vi "HEWH RLT PRAT.vi"() -> ()   [LabVIEW 2016] (continued)
        n576 = local read "Temp Decline Complete D"() -> (w1181:bool)
        n577 = call "HEWH Temperature Decline.vi"("Error In"=w1182, "Station"="D", "Temp Decline Complete A"=w1181, "Draw Parameters Seq"=w1185) -> ("Error Out"=w1180:errorcluster, "Output States"=w1184:string)  [unwired: 5 in, 1 out]
        n578 = call <vilib>:"Add State(s) to Queue__jki_lib_state_machine.vi"("State(s) in Front (\"\")"=w1184, "State(s) in (\"\")"=w1189) -> ("States Out"=w1188:string)  [unwired: 13 in]
      }
      frame "Set Draw Station" {
        n579 = case shown="\"D\"" w1197 {
          tunnel: w1196 -> [w1217 w1233 w1251 w1268]
          tunnel: [w1216 w1234 w1250 w1267] -> w1198
          tunnel: w1194 -> [w1213 w1230 w1245 w1264]
          tunnel: w1193 -> [w1210 _ _ _]
          tunnel: w1192 -> [_ w1227 _ _]
          tunnel: w1191 -> [_ _ w1244 _]
          tunnel: w1190 -> [_ _ _ w1261]
          frame "A", Default {
            n580 = Unbundle By Name(w1210) -> ("GEA2 Reference Out"=w1219:refnum<k24>, "GEA2 Event Registration"=w1218:refnum<event-registration>)
            n581 = Unbundle By Name(w1213) -> ("Draw Parameters Seq"=w1212:T41)
            n582 = Unbundle By Name(w1212) -> ("Station A.Mode Setting"=w1211:T15)
            n583 = call "HEWH_DSM_CMD.vi"("Heating Mode"=w1211, "GEA2 Commands and Requests"=GEA2_Commands."CMD_UPDATE_MODE") -> ("Input Data"=w1214:T74)  [unwired: 7 in, 1 out]
            n584 = for {
              N: 5 -> [_]
              tunnel: w1219 -> [w1225]
              tunnel: w1218 -> [w1224]
              tunnel: w1214 -> [w1221]
              shift-right: [w1222] -> w1216
              shift-left: w1217 -> [w1223]
              n585 = call "GEA2 Send and Receive Message.vi"("GEA2 Reference In"=w1225, "Input Data"=w1221, "GEA2 Event Registration"=w1224, "Error In"=w1223) -> ("Error Out"=w1222:errorcluster)  [unwired: 6 in, 5 out]
              n586 = Wait Until Next ms Multiple(millisecond multiple=u32 100) -> ()  [unwired: 1 out]
            }
          }
          frame "B" {
            n587 = Unbundle By Name(w1230) -> ("Draw Parameters Seq"=w1229:T41)
            n588 = Unbundle By Name(w1227) -> ("GEA2 Reference Out"=w1236:refnum<k24>, "GEA2 Event Registration"=w1235:refnum<event-registration>)
            n589 = Unbundle By Name(w1229) -> ("Station B.Mode Setting"=w1228:T15)
            n590 = call "HEWH_DSM_CMD.vi"("Heating Mode"=w1228, "GEA2 Commands and Requests"=GEA2_Commands."CMD_UPDATE_MODE") -> ("Input Data"=w1231:T74)  [unwired: 7 in, 1 out]
            n591 = for {
              N: 5 -> [_]
              tunnel: w1236 -> [w1242]
              tunnel: w1235 -> [w1241]
              tunnel: w1231 -> [w1238]
              shift-right: [w1240] -> w1234
              shift-left: w1233 -> [w1239]
              n592 = call "GEA2 Send and Receive Message.vi"("GEA2 Reference In"=w1242, "Input Data"=w1238, "GEA2 Event Registration"=w1241, "Error In"=w1239) -> ("Error Out"=w1240:errorcluster)  [unwired: 6 in, 5 out]
              n593 = Wait Until Next ms Multiple(millisecond multiple=u32 100) -> ()  [unwired: 1 out]
            }
          }
          frame "C" {
            n594 = Unbundle By Name(w1245) -> ("Draw Parameters Seq"=w1247:T41)
            n595 = Unbundle By Name(w1244) -> ("GEA2 Reference Out"=w1253:refnum<k24>, "GEA2 Event Registration"=w1252:refnum<event-registration>)
            n596 = Unbundle By Name(w1247) -> ("Station C.Mode Setting"=w1246:T15)
            n597 = call "HEWH_DSM_CMD.vi"("Heating Mode"=w1246, "GEA2 Commands and Requests"=GEA2_Commands."CMD_UPDATE_MODE") -> ("Input Data"=w1248:T74)  [unwired: 7 in, 1 out]
            n598 = for {
              N: 5 -> [_]
              tunnel: w1253 -> [w1259]
              tunnel: w1252 -> [w1258]
              tunnel: w1248 -> [w1255]
              shift-right: [w1256] -> w1250
              shift-left: w1251 -> [w1257]
              n599 = call "GEA2 Send and Receive Message.vi"("GEA2 Reference In"=w1259, "Input Data"=w1255, "GEA2 Event Registration"=w1258, "Error In"=w1257) -> ("Error Out"=w1256:errorcluster)  [unwired: 6 in, 5 out]
              n600 = Wait Until Next ms Multiple(millisecond multiple=u32 100) -> ()  [unwired: 1 out]
            }
          }
          frame "D" {
            n601 = Unbundle By Name(w1264) -> ("Draw Parameters Seq"=w1263:T41)
            n602 = Unbundle By Name(w1261) -> ("GEA2 Reference Out"=w1270:refnum<k24>, "GEA2 Event Registration"=w1269:refnum<event-registration>)
            n603 = Unbundle By Name(w1263) -> ("Station D.Mode Setting"=w1262:T15)
            n604 = call "HEWH_DSM_CMD.vi"("Heating Mode"=w1262, "GEA2 Commands and Requests"=GEA2_Commands."CMD_UPDATE_MODE") -> ("Input Data"=w1265:T74)  [unwired: 7 in, 1 out]
            n605 = for {
              N: 5 -> [_]
              tunnel: w1270 -> [w1276]
              tunnel: w1269 -> [w1275]
              tunnel: w1265 -> [w1272]
              shift-right: [w1273] -> w1267
              shift-left: w1268 -> [w1274]
              n606 = call "GEA2 Send and Receive Message.vi"("GEA2 Reference In"=w1276, "Input Data"=w1272, "GEA2 Event Registration"=w1275, "Error In"=w1274) -> ("Error Out"=w1273:errorcluster)  [unwired: 6 in, 5 out]
              n607 = Wait Until Next ms Multiple(millisecond multiple=u32 100) -> ()  [unwired: 1 out]
            }
          }
        }
        n608 = for {
          N: 10 -> [_]
          tunnel: w1197 -> [w1204]
          shift-right: [w1206] -> w1199
          shift-left: w1198 -> [w1205]
          n609 = Wait Until Next ms Multiple(millisecond multiple=u32 100) -> ()  [unwired: 1 out]
          n610 = call "UTILITY String Notifier.vi"("Status"=UTILITY_Notifier."Set", "error in (no error)"=w1205, "Set Status"=w1204, "name (unnamed)"="Draw Station") -> ("error out"=w1206:errorcluster)  [unwired: 6 in, 1 out]
        }
        n611 = call <vilib>:"Add State(s) to Queue__jki_lib_state_machine.vi"("State(s) in (\"\")"=w1202) -> ("States Out"=w1201:string)  [unwired: 14 in]
        "Draw Station" <- w1197
      }
      frame "-------Dispense Algorithm--------" {
        n612 = call <vilib>:"Add State(s) to Queue__jki_lib_state_machine.vi"("State(s) in (\"\")"=w1281) -> ("States Out"=w1280:string)  [unwired: 14 in]
      }
      frame "Dispense Gallons" {
        n613 = Unbundle By Name(w1311) -> ("Current Cond A"=w1286:T1, "Current Cond B"=w1285:T1, "Current Cond C"=w1284:T1, "Current Cond D"=w1283:T1, "Draw Parameters Seq.Station A.Flow Rate (GPM)"=→"GPM Target (Station A)":dbl, "Draw Parameters Seq.Station B.Flow Rate (GPM)"=→"GPM Target (Station B)":dbl, "Draw Parameters Seq.Station C.Flow Rate (GPM)"=→"GPM Target (Station C)":dbl, "Draw Parameters Seq.Station D.Flow Rate (GPM)"=→"GPM Target (Station D)":dbl, "Draw Parameters Seq.Station A.Temperature (F)"=→"Degree Setting( Station A)":dbl, "Draw Parameters Seq.Station B.Temperature (F)"=→"Degree Setting( Station B)":dbl, "Draw Parameters Seq.Station C.Temperature (F)"=→"Degree Setting( Station C)":dbl, "Draw Parameters Seq.Station D.Temperature (F)"=→"Degree Setting( Station D)":dbl, "Draw Parameters Seq.Station D.Condition Value #1"=w1296:dbl, "Draw Parameters Seq.Station C.Condition Value #1"=w1297:dbl, "Draw Parameters Seq.Station B.Condition Value #1"=w1298:dbl, "Draw Parameters Seq.Station A.Condition Value #1"=w1299:dbl, "Draw Parameters Seq.Station A.Terminate Condition"=w1295:T16, "Draw Parameters Seq.Station B.Terminate Condition"=w1294:T16, "Draw Parameters Seq.Station C.Terminate Condition"=w1293:T16, "Draw Parameters Seq.Station D.Terminate Condition"=w1291:T16, "Draw Parameters Seq"=w1292:T41)
        n614 = call "HEWH Update Draw Amount Display.vi"("Terminate Condition A"=w1295, "Terminate Condition B"=w1294, "Terminate Condition C"=w1293, "Terminate Condition D"=w1291, "Error In"=w1301, "Gallons to Draw A"=w1299, "Gallons to Draw B"=w1298, "Gallons to Draw C"=w1297, "Gallons to Draw D"=w1296) -> ("Draw Amount (Station A)"=→"Draw Amount (Station A)":dbl, "Draw Amount (Station B)"=→"Draw Amount (Station B)":dbl, "Draw Amount (Station C)"=→"Draw Amount (Station C)":dbl, "Draw Amount (Station D)"=→"Draw Amount (Station D)":dbl, "Error Out"=w1300:errorcluster)  [unwired: 6 in]
        n615 = flat-sequence {
          tunnel: [w1329] -> w1317
          tunnel: w1300 -> [w1328]
          tunnel: [w1328] -> w1316
          tunnel: w1314 -> [w1327]
          tunnel: [w1327] -> w1313
          tunnel: w1292 -> [w1326]
          tunnel: [w1325] -> w1310
          tunnel: w1286 -> [w1324]
          tunnel: w1285 -> [w1323]
          tunnel: w1284 -> [w1322]
          tunnel: w1283 -> [w1321]
          tunnel: [w1320] -> w1282
          tunnel: w1317 -> [w1361]
          tunnel: [w1365] -> w1315
          tunnel: w1316 -> [w1367]
          tunnel: w1313 -> [w1368]
          tunnel: [w1366] -> w1312
          tunnel: w1310 -> [w1360]
          tunnel: w1282 -> [w1359]
          frame #0 {
            n616 = local read "Draw Station"() -> (w1330:string)
            n617 = case shown="\"D\"" w1330 {
              tunnel: [Station_ID_Selector."A" ("Station ID") Station_ID_Selector."B" ("Station ID") Station_ID_Selector."C" ("Station ID") Station_ID_Selector."D" ("Station ID")] -> w1329
              tunnel: w1326 -> [w1336 w1343 w1350 w1355]
              tunnel: [w1334 w1342 w1349 w1358] -> w1325
              tunnel: w1324 -> [w1331 _ _ _]
              tunnel: w1323 -> [_ w1338 _ _]
              tunnel: w1322 -> [_ _ w1345 _]
              tunnel: w1321 -> [_ _ _ w1352]
              tunnel: [w1331 w1338 w1345 w1352] -> w1320
              frame "A", Default {
                n618 = Unbundle By Name(w1336) -> ("Station A"=w1335:T14)
                n619 = local read "Use Last Start Condition A?"() -> (w1333:bool)
                n620 = local read "Station A Test Sequence"() -> (w1332:T14[])
                n621 = call "HEWH Set Draw Station.vi"("Use Last Start Condition?"=w1333, "Station"=w1335, "Station Test Sequence"=w1332) -> ("Station Set"=w1334:T14)  [unwired: 7 in, 1 out]
              }
              frame "B" {
                n622 = local read "Use Last Start Condition B?"() -> (w1339:bool)
                n623 = local read "Station B Test Sequence"() -> (w1341:T14[])
                n624 = Unbundle By Name(w1343) -> ("Station B"=w1340:T14)
                n625 = call "HEWH Set Draw Station.vi"("Use Last Start Condition?"=w1339, "Station"=w1340, "Station Test Sequence"=w1341) -> ("Station Set"=w1342:T14)  [unwired: 7 in, 1 out]
              }
              frame "C" {
                n626 = local read "Station C Test Sequence"() -> (w1348:T14[])
                n627 = local read "Use Last Start Condition C?"() -> (w1346:bool)
                n628 = Unbundle By Name(w1350) -> ("Station C"=w1347:T14)
                n629 = call "HEWH Set Draw Station.vi"("Use Last Start Condition?"=w1346, "Station"=w1347, "Station Test Sequence"=w1348) -> ("Station Set"=w1349:T14)  [unwired: 7 in, 1 out]
              }
              frame "D" {
                n630 = local read "Use Last Start Condition D?"() -> (w1353:bool)
                n631 = Unbundle By Name(w1355) -> ("Station D"=w1354:T14)
                n632 = local read "Station D Test Sequence"() -> (w1356:T14[])
                n633 = call "HEWH Set Draw Station.vi"("Use Last Start Condition?"=w1353, "Station"=w1354, "Station Test Sequence"=w1356) -> ("Station Set"=w1358:T14)  [unwired: 7 in, 1 out]
              }
            }
          }
          frame #1 {
            n634 = Bundle By Name(cluster=T54 {"Start Draw"=FALSE, "Station ID"=enum."A", "Station Draw Info"={"Sequence #"=0.0, "Cycles"=0, "Mode Setting"="", "Flow Rate (GPM)"=0.0, "Temperature (F)"=0.0, "Reset Timer"=FALSE, "Use Temp Decline Method"=FALSE, "Terminate Condition"=enum."C1-Terminate Draw @ Gallon Mark", "Condition Value #1"=0.0, "UE"=FALSE, "LE"=FALSE, "Comp"=FALSE, "Fan"=FALSE, "Test End Time (Sec)"=0.0, "Purge Until Cutout"=FALSE, "Start Conditions"=enum."Heat Source Cutout", "Condition Value #2"=0.0, "Remove Power"=FALSE, "Time"=0.0, "Check Special Cond."=enum."SC2-Check Heat Source (On-C2/Off-C1)", "Condition#"=enum."C1", "Draw Flags"=enum."N/A", "Data Processing Delay (FHD 15sec, UEF 5 Sec)"=0.0, "Test Complete"=FALSE}, "Send Condition"=enum."N/A"}, "Send Condition"=w1359, "Start Draw"=TRUE, "Station ID"=w1361, "Station Draw Info"=w1360) -> (w1362:T54)
            n635 = Enqueue Element(queue=w1368, element=w1362, error in (no error)=w1367) -> (queue out=w1366:refnum<queue>, error out=w1365:errorcluster)  [unwired: 1 in, 1 out]
            "Station Draw Info" <- w1360
          }
        }
        n636 = call <vilib>:"Add State(s) to Queue__jki_lib_state_machine.vi"("State(s) in (\"\")"=w1319) -> ("States Out"=w1318:string)  [unwired: 14 in]
      }
    }
    n637 = case shown="False" "Debug" {
      tunnel: [w230 w233] -> w220
      tunnel: w219 -> [w230 w232]
      tunnel: w217 -> [_ w231]
      frame False {
      }
      frame True {
        n638 = Build Array (concatenate)(w232, w231) -> (w233:string[])
      }
    }
    "Main Control" <- w220
    "MainLoop" <- w211
  }
  "Finish" <- w128
  n639 = Unbundle By Name(w61) -> ("GEA2 Reference Out"=w42:refnum<k24>, "GEA2 Event Registration"=w41:refnum<event-registration>)
  n640 = Unbundle By Name(w62) -> ("GEA2 Reference Out"=w43:refnum<k24>, "GEA2 Event Registration"=w40:refnum<event-registration>)
  n641 = Unbundle By Name(w46) -> ("GEA2 Reference Out"=w44:refnum<k24>, "GEA2 Event Registration"=w39:refnum<event-registration>)
  n642 = Unbundle By Name(w47) -> ("GEA2 Reference Out"=w45:refnum<k24>, "GEA2 Event Registration"=w38:refnum<event-registration>)
  n643 = while "Data Acquisition Steps" {
    shift-right: [w1390] -> _
    shift-left: _ -> [w1389]
    shift-right: [w1393] -> w120
    shift-left: _ -> [w1388]
    shift-right: [w1392] -> _
    shift-left: w123 -> [w1394]
    tunnel: w78 -> [w1387]
    tunnel: w86 -> [w1386]
    shift-right: [w1382] -> _
    shift-left: string[] [] -> [w1385]
    tunnel: w52 -> [w1381]
    tunnel: w47 -> [w1380]
    tunnel: w46 -> [w1379]
    tunnel: w62 -> [w1378]
    tunnel: w61 -> [w1377]
    tunnel: w51 -> [w1376]
    tunnel: w50 -> [w1375]
    tunnel: w49 -> [w1374]
    tunnel: w48 -> [w1373]
    tunnel: w22 -> [w1372]
    tunnel: w21 -> [w1371]
    tunnel: w20 -> [w1370]
    tunnel: w19 -> [w1369]
    stop <- w1391 stop-if-true
    # "Data Acquisition Steps"
    n644 = call <vilib>:"Parse State Queue__JKI_lib_State_Machine.vi"("State Queue"=w1394, "Error In (no error)"=w1388) -> ("Remaining States"=w1396:string, "Current State"=w1384:string, "Arguments"=w1395:string)  [unwired: 11 in]
    "DAQ State" <- w1384
    n645 = case shown="\"Data: Get GEA2 A\"" w1384 {
      selector: w1384 -> [_ w1523 _ _ _ _ _ _ _ _ _ _ _ _ _ _ _ _ _ _ _ _ _ _ _ _ _ _ _ _ _ _ _ _ _ _ _ _ _ _ _ _ _ _ _]
      tunnel: w1396 -> [w1416 w1526 w1538 w1546 w1558 w1588 w1637 w1656 w1675 w1694 w1713 w1723 w1751 w1759 w1799 w1807 w1838 w1883 w1922 w1961 w2000 w2033 w2064 w2095 w2126 w2152 w2197 w2247 w2270 w2279 w2309 w2339 w2368 w2421 w2454 w2482 w2510 w2538 w2575 w2590 w2614 w2638 w2662 w2673 w2695]
      tunnel: w1395 -> [_ _ _ _ _ _ _ _ _ _ _ _ _ _ _ _ _ _ _ _ _ _ _ _ _ _ _ _ _ _ _ _ _ _ _ _ _ _ _ _ _ _ _ _ _]
      tunnel: [w1414 w1528 errorcluster {"status"=FALSE, "code"=0, "source"=""} ("error out") w1542 w1556 w1561 w1616 w1639 w1658 w1677 w1696 w1721 w1747 w1756 w1790 w1805 w1831 w1872 w1913 w1952 w1991 w2011 w2045 w2072 w2107 w2140 w2182 w2232 w2262 w2276 w2305 w2335 w2364 w2404 w2434 w2480 w2508 w2536 w2573 w2581 w2605 w2629 w2653 w2674 w2686] -> w1393
      tunnel: w1388 -> [w1411 w1527 w1534 w1543 w1556 w1561 w1626 w1640 w1659 w1678 w1697 w1721 w1748 w1757 w1793 w1805 w1812 w1874 w1915 w1954 w1993 w2022 w2057 w2088 w2119 w2148 w2183 w2233 w2263 w2277 w2306 w2336 w2365 w2413 w2434 w2480 w2508 w2536 w2573 w2577 w2601 w2625 w2650 w2674 w2687]
      tunnel: [w1415 w1525 w1537 w1545 w1557 w1587 w1636 w1655 w1674 w1693 w1712 w1722 w1750 w1758 w1798 w1806 w1837 w1882 w1921 w1960 w1999 w2034 w2065 w2096 w2127 w2151 w2196 w2246 w2269 w2278 w2308 w2338 w2367 w2420 w2453 w2481 w2509 w2537 w2574 w2589 w2613 w2637 w2661 w2673 w2695] -> w1392
      tunnel: [_ _ _ w1540 _ _ _ _ _ _ _ _ _ _ _ _ _ _ _ _ _ _ _ _ _ _ _ _ _ _ _ _ _ _ _ _ _ _ _ _ _ _ _ _ _] -> w1391
      tunnel: [w1413 w1522 w1533 w1544 w1555 w1572 w1631 w1654 w1673 w1692 w1711 w1714 w1737 w1755 w1797 w1804 w1836 w1881 w1920 w1959 w1998 w2032 w2063 w2094 w2125 w2150 w2195 w2245 w2264 w2275 w2304 w2334 w2363 w2419 w2448 w2473 w2499 w2529 w2572 w2583 w2606 w2630 w2654 w2672 w2675] -> w1390
      tunnel: w1389 -> [w1412 w1522 w1533 w1544 w1555 _ w1632 w1654 w1673 w1692 w1711 w1715 w1742 w1755 w1797 w1804 w1833 w1878 w1919 w1958 w1997 w2031 w2062 w2093 w2124 w2139 w2190 w2240 w2264 w2273 w2307 w2337 w2366 w2419 w2449 w2474 w2500 w2530 w2571 w2584 w2607 w2631 w2655 w2672 w2675]
      tunnel: w1387 -> [_ _ _ _ _ _ w1625 _ _ _ _ _ _ _ w1792 _ _ w1873 w1914 w1953 w1992 _ _ _ _ _ _ _ _ _ _ _ _ _ _ _ _ _ _ _ _ _ _ _ _]
      tunnel: w1386 -> [w1410 _ _ _ _ _ _ _ _ _ _ _ _ _ _ _ _ _ _ _ _ _ _ _ _ _ _ _ _ _ _ _ _ _ _ _ _ _ _ _ _ _ _ _ _]
      tunnel: w1381 -> [_ _ _ _ _ _ _ _ _ _ _ _ _ _ _ _ w1829 _ _ _ _ _ _ _ _ _ _ _ _ _ _ _ _ _ _ _ _ _ _ _ _ _ _ _ _]
      tunnel: w1380 -> [_ _ _ _ _ _ _ w1643 _ _ _ _ _ _ _ _ _ _ _ _ _ w2025 _ _ _ _ _ _ _ _ _ _ _ _ _ _ _ _ _ _ _ _ _ _ _]
      tunnel: w1379 -> [_ _ _ _ _ _ _ _ w1662 _ _ _ _ _ _ _ _ _ _ _ _ _ w2053 _ _ _ _ _ _ _ _ _ _ _ _ _ _ _ _ _ _ _ _ _ _]
      tunnel: w1378 -> [_ _ _ _ _ _ _ _ _ w1681 _ _ _ _ _ _ _ _ _ _ _ _ _ w2084 _ _ _ _ _ _ _ _ _ _ _ _ _ _ _ _ _ _ _ _ _]
      tunnel: w1377 -> [_ _ _ _ _ _ _ _ _ _ w1700 _ _ _ _ _ _ _ _ _ _ _ _ _ w2115 _ _ _ _ _ _ _ _ _ _ _ _ _ _ _ _ _ _ _ _]
      tunnel: w1376 -> [_ _ _ _ _ _ _ _ _ _ _ _ _ _ _ _ _ _ _ _ _ _ _ _ _ _ _ _ _ w2272 _ _ _ _ _ _ _ _ _ _ _ _ _ _ _]
      tunnel: w1375 -> [_ _ _ _ _ _ _ _ _ _ _ _ _ _ _ _ _ _ _ _ _ _ _ _ _ _ _ _ _ _ w2302 _ _ _ _ _ _ _ _ _ _ _ _ _ _]
      tunnel: w1374 -> [_ _ _ _ _ _ _ _ _ _ _ _ _ _ _ _ _ _ _ _ _ _ _ _ _ _ _ _ _ _ _ w2332 _ _ _ _ _ _ _ _ _ _ _ _ _]
      tunnel: w1373 -> [_ _ _ _ _ _ _ _ _ _ _ _ _ _ _ _ _ _ _ _ _ _ _ _ _ _ _ _ _ _ _ _ w2361 _ _ _ _ _ _ _ _ _ _ _ _]
      tunnel: w1372 -> [_ _ _ _ _ _ _ _ _ _ _ w1720 _ _ _ _ _ _ _ _ _ _ _ _ _ _ _ _ _ _ _ _ _ _ _ _ _ _ _ _ _ _ _ _ _]
      tunnel: w1371 -> [_ _ _ _ _ _ _ _ _ _ _ w1719 _ _ _ _ _ _ _ _ _ _ _ _ _ _ _ _ _ _ _ _ _ _ _ _ _ _ _ _ _ _ _ _ _]
      tunnel: w1370 -> [_ _ _ _ _ _ _ _ _ _ _ w1718 _ _ _ _ _ _ _ _ _ _ _ _ _ _ _ _ _ _ _ _ _ _ _ _ _ _ _ _ _ _ _ _ _]
      tunnel: w1369 -> [_ _ _ _ _ _ _ _ _ _ _ w1717 _ _ _ _ _ _ _ _ _ _ _ _ _ _ _ _ _ _ _ _ _ _ _ _ _ _ _ _ _ _ _ _ _]
      frame "", "Idle" {
        n646 = call "UTILITY JKI Loop Timer.vi"("PID gains"="PID gains", "Use Fuzzy Logic"="Use Fuzzy Logic", "Initialize Rate"="Initialize Rate", "K(0.3)"="K(0.2)", "Scan Rate (Seconds)"="Scan Rate (Seconds)") -> ("Rate"=→"Rate":dbl, "New Time"=w1404:dbl)  [unwired: 5 in]
        n647 = Multiply(x=T10 1000.0 ("y"), y=w1404) -> (x*y=w1403:T10)
        n648 = event shown="[2] <Update  Cal and Calib DAQ>: User Event" {
          selector: w1410 -> [_ _ _ _]
          dyn-events: _ -> [_ _ _ _]
          timeout: w1403 -> [_ _ _ _]
          tunnel: w1416 -> [w1433 w1441 w1455 w1456]
          tunnel: [w1432 w1442 w1455 w1457] -> w1415
          tunnel: w1412 -> [w1428 w1443 w1449 w1459]
          tunnel: [w1429 w1439 w1454 w1460] -> w1414
          tunnel: w1411 -> [w1429 w1439 w1454 w1461]
          tunnel: [w1428 w1443 w1448 w1464] -> w1413
          event Timeout {
            n649 = event-data() -> ()  [unwired: 1 in, 1 out]
            n650 = Unbundle By Name(w1428) -> ("Core HEWH Data Input A.LV Program"=w1427:T24)
            n651 = case shown="\"PRAT\", \"HEWH RLT\"" w1427 {
              tunnel: [w1435 "Data: Get Time\nData: Get MW100 (Station A)\nData: Get MW100 (Station B)\nData: Get MW100 (Station C)\nData: Get MW100 (Station D)\nData: Get GEA2 A\nData: Get GEA2 B\nData: Get GEA2 C\nData: Get GEA2 D\nData: Get Agilent\nGet Temp and Humidity\nData: Check Errors\nData: Update RLT Channels\nShow Data A\nShow Data B\nShow Data C\nShow Data D\nCalculate Max AVG TC Temp"] -> w1431
              tunnel: "Get Gas Data" -> [w1434 _]
              frame "HEWH", Default {
                n652 = case shown="False" w1434 {
                  tunnel: ["Data: Get Time\nData: Get MW100 (Station A)\nData: Get GEA2 A\nData: Get Agilent\nGet Temp and Humidity\nData: Update RLT Channels\nShow Data A\nCalculate Max AVG TC Temp" "Data: Get Time\nData: Get MW100 (Station A)\nData: Get GEA2 A\nData: Get Agilent\nGet Temp and Humidity\nGet Gas Data\nData: Update RLT Channels\nShow Data A\nCalculate Max AVG TC Temp"] -> w1435
                  frame False {
                  }
                  frame True {
                  }
                }
              }
              frame "PRAT", "HEWH RLT" {
              }
            }
            n653 = local read "Final Headers B"() -> (w1419:bool)
            n654 = local read "Log Data Output (D)"() -> (w1423:bool)
            n655 = local read "Log Data Output (C)"() -> (w1424:bool)
            n656 = local read "Final Headers A"() -> (w1420:bool)
            n657 = local read "Final Headers C"() -> (w1418:bool)
            n658 = local read "Log Data Output (A)"() -> (w1426:bool)
            n659 = local read "Log Data Output (B)"() -> (w1425:bool)
            n660 = local read "Final Headers D"() -> (w1417:bool)
            n661 = call "HEWH Create Save Data States.vi"("LV Program"=w1427, "Data Loop?"=TRUE, "Final Headers A"=w1420, "Final Headers C"=w1418, "Log Data Output (C)"=w1424, "Log Data Output (A)"=w1426, "Log Data Output (D)"=w1423, "Log Data Output (B)"=w1425, "Final Headers B"=w1419, "Final Headers D"=w1417) -> ("SM States"=w1430:string)  [unwired: 8 in, 1 out]
            n662 = call <vilib>:"Add State(s) to Queue__jki_lib_state_machine.vi"("State(s) in Front (\"\")"=w1431, "State(s) in (\"\")"=w1433, "State(s) at Back (\"\")"=w1430) -> ("States Out"=w1432:string)  [unwired: 12 in]
          }
          event "Finish": Value Change {
            n663 = event-data() -> ()  [unwired: 1 in, 6 out]
            n664 = call <vilib>:"Add State(s) to Queue__jki_lib_state_machine.vi"("State(s) in Front (\"\")"="Shutdown Equipment\nExit", "State(s) in (\"\")"=w1441) -> ("States Out"=w1442:string)  [unwired: 13 in]
          }
          event User Event {
            n665 = event-data() -> ()  [unwired: 1 in, 5 out]
            n666 = local read "Station A Update"() -> (w1450:T12)
            n667 = local read "Station B Update"() -> (w1451:T12)
            n668 = local read "Station C Update"() -> (w1452:T12)
            n669 = local read "Station D Update"() -> (w1453:T12)
            n670 = Unbundle By Name(w1450) -> ("Calc and Calibration"=w1447:T23)
            n671 = Unbundle By Name(w1451) -> ("Calc and Calibration"=w1446:T23)
            n672 = Unbundle By Name(w1452) -> ("Calc and Calibration"=w1445:T23)
            n673 = Unbundle By Name(w1453) -> ("Calc and Calibration"=w1444:T23)
            n674 = Bundle By Name(cluster=w1449, "Core HEWH Data Input A.Calc and Calibration"=w1447, "Core HEWH Data Input B.Calc and Calibration"=w1446, "Core HEWH Data Input C.Calc and Calibration"=w1445, "Core HEWH Data Input D.Calc and Calibration"=w1444) -> (w1448:T80)
          }
          event User Event {
            n675 = event-data() -> ()  [unwired: 1 in, 5 out]
            n676 = local read "Station ID to Reset"() -> (w1465:T25)
            n677 = case shown="\"A\", Default" w1465 {
              tunnel: w1459 -> [w1479 w1493 w1507 w1521]
              tunnel: [w1478 w1492 w1506 w1520] -> w1464
              tunnel: [w1476 w1484 w1498 w1511] -> w1462
              tunnel: w1461 -> [w1475 w1486 w1505 w1519]
              tunnel: [w1474 w1485 w1504 w1518] -> w1460
              tunnel: w1459 -> [w1472 w1491 w1502 w1517]
              frame "A", Default {
                n678 = Unbundle By Name(w1472) -> ("Core HEWH Data Input A.Calc and Calibration"=w1470:T23)
                n679 = local read "Log Data Output (A)"() -> (w1477:bool)
                n680 = local read "Updated File Path A"() -> (w1473:T2)
                n681 = local read "Reset Cycle Count"() -> (w1468:bool)
                n682 = call "HEWH Final Data Check.vi"("Station Message"="MessageA", "Input State"="Add Final Data A", "Calc and Calibration in"=w1470, "error in (no error)"=w1475, "Reset Cycle Count"=w1468, "Updated File Path A in"=w1473, "Log Data Output (A)"=w1477) -> ("error out"=w1474:errorcluster, "Updated File Path A out"=w1471:T2, "Calc and Calibration out"=w1469:T23, "Output State"=w1476:string)  [unwired: 1 in]
                n683 = Bundle By Name(cluster=w1479, "Core HEWH Data Input A.Calc and Calibration"=w1469, "File Locations A"=w1471) -> (w1478:T80)
              }
              frame "B" {
                n684 = Unbundle By Name(w1491) -> ("Core HEWH Data Input B.Calc and Calibration"=w1490:T23)
                n685 = local read "Log Data Output (B)"() -> (w1489:bool)
                n686 = local read "Updated File Path B"() -> (w1488:T2)
                n687 = local read "Reset Cycle Count"() -> (w1487:bool)
                n688 = call "HEWH Final Data Check.vi"("Station Message"="MessageB", "Input State"="Add Final Data B" ("State(s) in Front (\"\")"), "Calc and Calibration in"=w1490, "error in (no error)"=w1486, "Reset Cycle Count"=w1487, "Updated File Path A in"=w1488, "Log Data Output (A)"=w1489) -> ("error out"=w1485:errorcluster, "Updated File Path A out"=w1481:T2, "Calc and Calibration out"=w1482:T23, "Output State"=w1484:string)  [unwired: 1 in]
                n689 = Bundle By Name(cluster=w1493, "Core HEWH Data Input B.Calc and Calibration"=w1482, "File Locations B"=w1481) -> (w1492:T80)
              }
              frame "C" {
                n690 = Unbundle By Name(w1502) -> ("Core HEWH Data Input C.Calc and Calibration"=w1501:T23)
                n691 = local read "Log Data Output (C)"() -> (w1503:bool)
                n692 = local read "Updated File Path C"() -> (w1500:T2)
                n693 = local read "Reset Cycle Count"() -> (w1497:bool)
                n694 = call "HEWH Final Data Check.vi"("Station Message"="MessageC", "Input State"="Add Final Data C" ("State(s) in Front (\"\")"), "Calc and Calibration in"=w1501, "error in (no error)"=w1505, "Reset Cycle Count"=w1497, "Updated File Path A in"=w1500, "Log Data Output (A)"=w1503) -> ("error out"=w1504:errorcluster, "Updated File Path A out"=w1495:T2, "Calc and Calibration out"=w1496:T23, "Output State"=w1498:string)  [unwired: 1 in]
                n695 = Bundle By Name(cluster=w1507, "Core HEWH Data Input C.Calc and Calibration"=w1496, "File Locations C"=w1495) -> (w1506:T80)
              }
              frame "D" {
                n696 = Unbundle By Name(w1517) -> ("Core HEWH Data Input D.Calc and Calibration"=w1516:T23)
                n697 = local read "Log Data Output (D)"() -> (w1515:bool)
                n698 = local read "Updated File Path D"() -> (w1514:T2)
                n699 = local read "Reset Cycle Count"() -> (w1513:bool)
                n700 = call "HEWH Final Data Check.vi"("Station Message"="MessageD", "Input State"="Add Final Data D" ("State(s) in Front (\"\")"), "Calc and Calibration in"=w1516, "error in (no error)"=w1519, "Reset Cycle Count"=w1513, "Updated File Path A in"=w1514, "Log Data Output (A)"=w1515) -> ("error out"=w1518:errorcluster, "Updated File Path A out"=w1509:T2, "Calc and Calibration out"=w1510:T23, "Output State"=w1511:string)  [unwired: 1 in]
                n701 = Bundle By Name(cluster=w1521, "Core HEWH Data Input D.Calc and Calibration"=w1510, "File Locations D"=w1509) -> (w1520:T80)
              }
            }
            n702 = call <vilib>:"Add State(s) to Queue__jki_lib_state_machine.vi"("State(s) in Front (\"\")"=w1462, "State(s) in (\"\")"=w1456) -> ("States Out"=w1458:string)  [unwired: 13 in]
            n703 = call <vilib>:"Add State(s) to Queue__jki_lib_state_machine.vi"("State(s) in Front (\"\")"="Data: Update RLT Channels" ("State(s) in Front (\"\")"), "State(s) in (\"\")"=w1458) -> ("States Out"=w1457:string)  [unwired: 13 in]
          }
        }
      }
      frame Default {
